vi "Mark10 Home Speed.vi"(11 "Speed":dbl) -> (3 "Cmds":string[](array[string]))   [LabVIEW 2015]
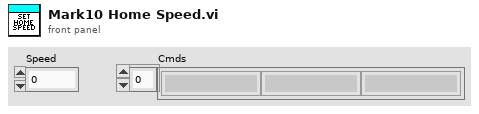
[diagram p1: front panel]
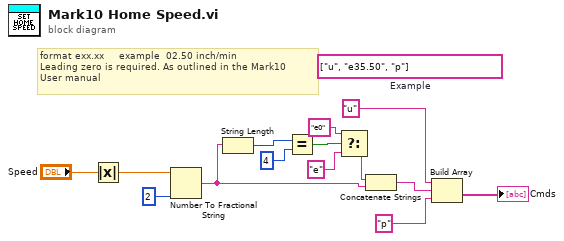
[diagram p0: block diagram]
diagram:
  (unwired) string[] ["u", "e35.50", "p"]  # Example
  # "format exx.xx     example  02.50 inch/min\nLeading zero is required. As outlined in the Mark10\nUser manual"
  n1 = Absolute Value(x="Speed") -> (abs(x)=w11:dbl)
  n2 = Number To Fractional String(number=w11, precision (6)=i16 2 ("width (-)")) -> (F-format string=w8:string)  [unwired: 2 in]
  n3 = String Length(string=w8) -> (length=w7:i32)
  n4 = Equal?(x=w7, y=4) -> (x = y?=w4:bool)
  n5 = Select(t="e0", s=w4, f="e") -> (s? t:f=w1:string)
  n6 = Concatenate Strings(w1, w8) -> (w10:string)
  n7 = Build Array("u", w10, "p") -> (→"Cmds":string[])
